vi "Get External Result Ref.vi"(11 "Test Run Result":refnum<class "Test Run Result.lvclass">) -> (3 "External Result Ref":string)   [LabVIEW 2026, in "Test Run Result.lvclass"]
uses:
  Test Run Result.lvclass
  Test Run Result.lvclass/Test Run Result.ctl
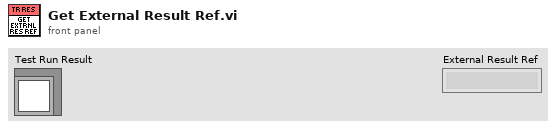
[diagram p1: front panel]
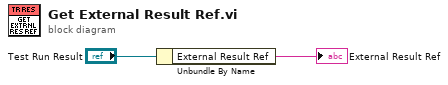
[diagram p0: block diagram]
diagram:
  n1 = Unbundle By Name("Test Run Result") -> ("External Result Ref"=→"External Result Ref":string)
